vi "Test SUBSCRIBE packet.vi"() -> ()   [LabVIEW 2013]
uses:
  source/Control Packets/SUBSCRIBE/SUBSCRIBE.lvclass
  source/Control Packets/SUBSCRIBE/Topic Subscription -- cluster.ctl
  source/Control Packets/ControlPacket/QualityOfService -- enum.ctl
  source/Control Packets/ControlPacket/ControlPacket.lvclass/ControlPacket.ctl
  source/Control Packets/ControlPacket/ControlPacket.lvclass
panel:
  out "Subscription Payload":bool
  out "Packet ID":u16 format="%04x"
  out "error out":errorcluster
  out "Packet Identifier":bool
  out "Packet type":bool
  out "All packets consumed":bool
  out "Complete Packet":bool
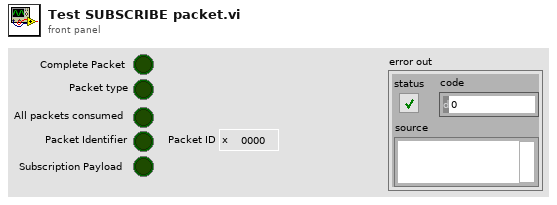
[diagram p1: front panel]
types:
  T1 = typedef "SUBSCRIBE.lvclass/Topic Subscription -- cluster.ctl" = cluster{"Topic Filter":string, "QoS":T2}
  T2 = typedef "ControlPacket.lvclass/QualityOfService -- enum.ctl" = enum16{"0 (At Most Once)", "1 (At Least Once)", "2 (Exactly Once)"}
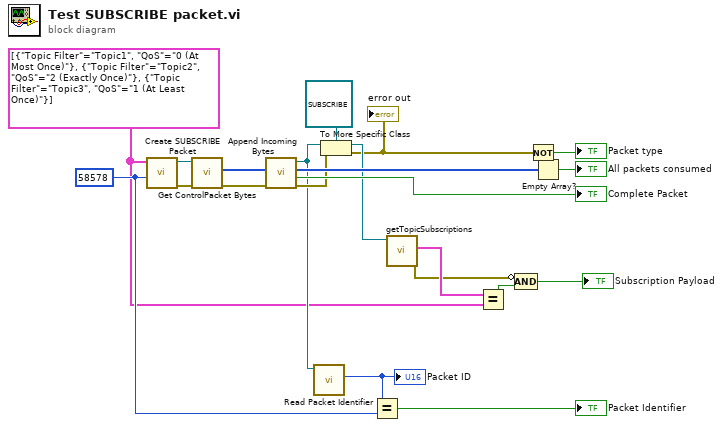
[diagram p0: block diagram]
diagram:
  w7 = T1[] [{"Topic Filter"="Topic1", "QoS"=enum."0 (At Most Once)"}, {"Topic Filter"="Topic2", "QoS"=enum."2 (Exactly Once)"}, {"Topic Filter"="Topic3", "QoS"=enum."1 (At Least Once)"}] ("Topic Subscriptions")
  w8 = u16 58578 ("Packet ID")
  n1 = call "Create SUBSCRIBE Packet.vi"("Packet ID"=w8, "Topic Subscriptions"=w7) -> ("error out"=w9:errorcluster, "SUBSCRIBE out"=w10:refnum<class "SUBSCRIBE.lvclass">)  [unwired: 8 in]
  n2 = call "Get ControlPacket Bytes.vi"("error in (no error)"=w9, "ControlPacket"=w10) -> ("error out"=w16:errorcluster, "Bytes Stream"=w21:u8[])  [unwired: 7 in, 1 out]
  n3 = call "Append Incoming Bytes.vi"("error in (no error)"=w16, "Incoming Packets"=w21) -> ("error out"=w15:errorcluster, "Complete Packet"=→"Complete Packet":bool, "Remaining Packets"=w19:u8[], "ControlPacket"=w12:refnum<class "ControlPacket.lvclass">)  [unwired: 6 in]
  n4 = call "Read Packet Identifier.vi"("ControlPacket in"=w12) -> ("Packet Identifier"=w14:u16)  [unwired: 9 in, 1 out]
  "Packet ID" <- w14
  n5 = To More Specific Class(target class=refnum<class "SUBSCRIBE.lvclass"> refnum ("SUBSCRIBE.lvclass"), reference=w12, error in=w15) -> (specific class reference=w6:refnum<class "SUBSCRIBE.lvclass">, error out=w5:errorcluster)
  "error out" <- w5
  n6 = Equal?(x=w14, y=w8) -> (x = y?=→"Packet Identifier":bool)
  n7 = call "getTopicSubscriptions.vi"("SUBSCRIBE in"=w6) -> ("error out"=w3:errorcluster, "Topic Subscriptions"=w4:T1[])  [unwired: 8 in, 1 out]
  n8 = Equal?(x=w4, y=w7) -> (x = y?=w2:bool)
  n9 = Compound Arithmetic op=AND(invert w3, w2) -> (→"Subscription Payload":bool)
  n10 = Not(x=w5) -> (.not. x?=→"Packet type":bool)
  n11 = Empty Array?(array=w19) -> (empty?=→"All packets consumed":bool)
